vi "WriteState.vi"(8 "Error In":errorcluster, 10 "State":bool, 11 "object in":refnum<class "Flipflop.lvclass">) -> (0 "Error Out":errorcluster, 3 "object out":refnum<class "Flipflop.lvclass">)   [LabVIEW 2021, in "Flipflop.lvclass"]
uses:
  Flipflop.lvclass
  Flipflop.lvclass/Flipflop.ctl
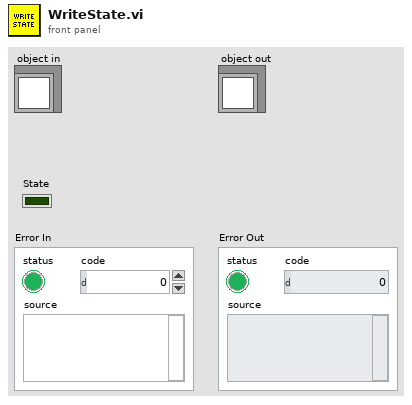
[diagram p1: front panel]
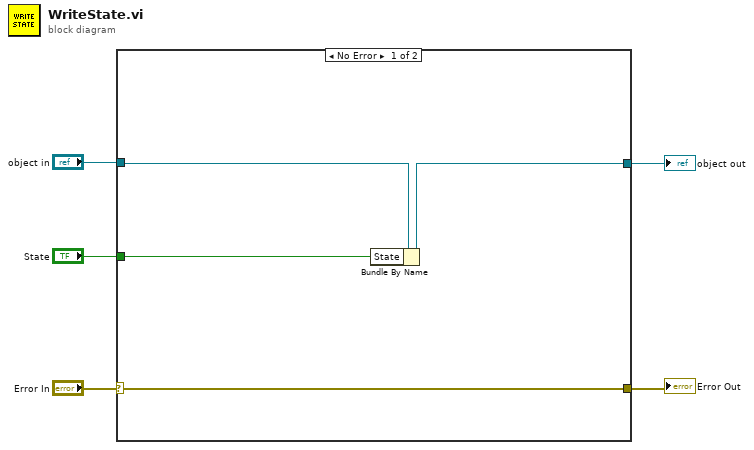
[diagram p0: block diagram]
diagram:
  n1 = case shown="No Error" "Error In" {
    selector: "Error In" -> [w8 w11]
    tunnel: [w8 w11] -> w4
    tunnel: [w6 w10] -> w2
    tunnel: "object in" -> [w7 w10]
    tunnel: "State" -> [w9 _]
    frame No Error {
      n2 = Bundle By Name(cluster=w7, "State"=w9) -> (w6:refnum<class "Flipflop.lvclass">)
    }
    frame Error {
    }
  }
  "Error Out" <- w4
  "object out" <- w2
